vi "Configure Channel (mA Normal).vi"(0 "VISA resource name":refnum<visa-resource-name>, 5 "Channel (0001)":string="0001", 7 "Enable Channel (True)":bool=TRUE, 9 "Span":T1={"mA Range (0 : 0-20mA)"=0, "Enable Span (False)"=FALSE, "Lower Span (0.0000)"=0.0, "Upper Span (20.0000)"=20.0, "Bias (0)"=0.0} {"mA Range (0 : 0-20mA)" items=["0-20mA"]; "Bias (0)" format="%_6g"; "Upper Span (20.0000)" step=0.001 format="%.3g"; "Lower Span (0.0000)" step=0.001 format="%.3g"}, 11 "error in (no error)":errorcluster) -> (4 "VISA resource name out":refnum<visa-resource-name>, 6 "Channel":string, 15 "error out":errorcluster)   [LabVIEW 2020, in "Yokogawa GX Series.lvlib"]
doc: "Sets the input range as voltage.\n\nCommand: SRangeAI"
uses:
  <instrlib>/Yokogawa GX Series/Yokogawa GX Series.lvlib
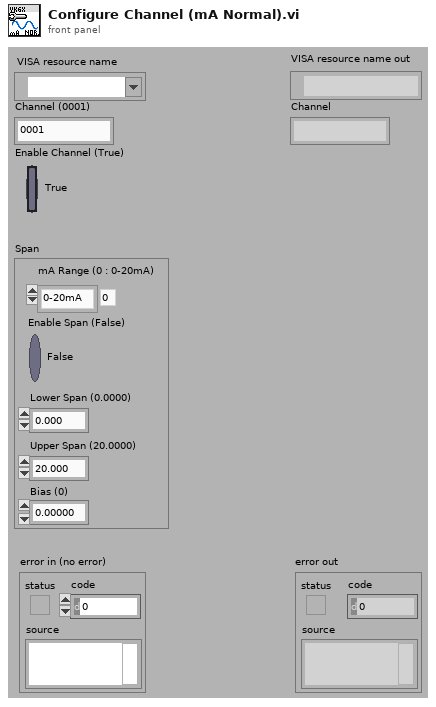
[diagram p1: front panel]
types:
  T1 = cluster{"mA Range (0 : 0-20mA)":i32, "Enable Span (False)":bool, "Lower Span (0.0000)":dbl, "Upper Span (20.0000)":dbl, "Bias (0)":dbl}
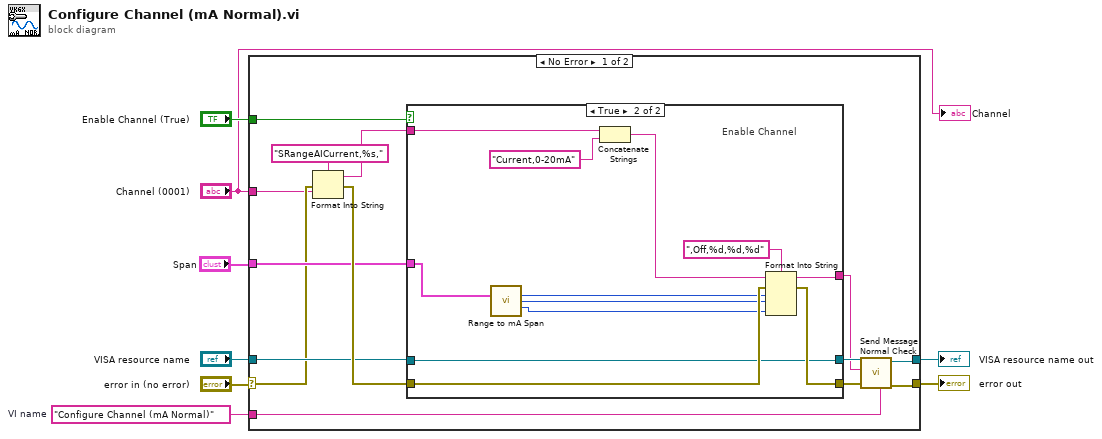
[diagram p0: block diagram]
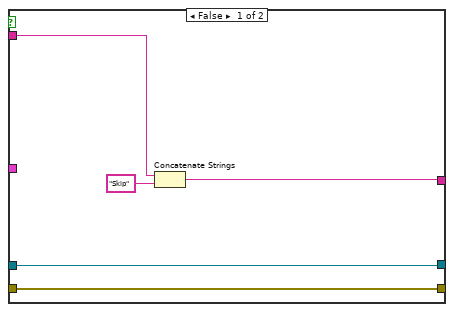
[diagram p2: hidden frame]
diagram:
  w4 = "Configure Channel (mA Normal)"  # VI name
  n1 = case shown="No Error" "error in (no error)" {
    selector: "error in (no error)" -> [w10 w40]
    tunnel: "Enable Channel (True)" -> [w19 _]
    tunnel: "VISA resource name" -> [w18 w41]
    tunnel: [w15 w41] -> w6
    tunnel: [w14 w40] -> w5
    tunnel: w4 -> [w13 _]
    tunnel: "Span" -> [w11 _]
    tunnel: "Channel (0001)" -> [w9 _]
    frame No Error {
      n2 = Format Into String(format string="SRangeAICurrent,%s,", error in=w10, w9) -> (resulting string=w20:string, error out=w21:errorcluster)  [unwired: 1 in]
      n3 = case shown="True" w19 {
        tunnel: w21 -> [w24 w34]
        tunnel: [w24 w38] -> w16
        tunnel: w20 -> [w25 w37]
        tunnel: [w27 w36] -> w12
        tunnel: w18 -> [w23 w33]
        tunnel: [w23 w33] -> w17
        tunnel: w11 -> [_ w31]
        frame False {
          n4 = Concatenate Strings(w25, "Skip") -> (w27:string)
        }
        frame True {
          # "Enable Channel"
          n5 = call <instrlib>:"Range to mA Span.vi"("Span"=w31) -> ("Lower Span"=w30:i32, "Upper Span"=w29:i32, "Bias"=w28:i32)  [unwired: 12 in]
          n6 = Concatenate Strings(w37, "Current,0-20mA") -> (w32:string)
          n7 = Format Into String(format string=",Off,%d,%d,%d", initial string=w32, error in=w34, w30, w29, w28) -> (resulting string=w36:string, error out=w38:errorcluster)
        }
      }
      n8 = call <instrlib>:"Send Message Normal Check.vi"("Source (\"\")"=w13, "error in (no error)"=w16, "Send Message (\"\")"=w12, "VISA resource name"=w17) -> ("error out"=w14:errorcluster, "VISA resource name out"=w15:refnum<visa-resource-name>)  [unwired: 2 in, 4 out]
    }
    frame Error {
    }
  }
  "error out" <- w5
  "VISA resource name out" <- w6
  "Channel" <- "Channel (0001)"
